vi "Initialize-panes.vi"(8 "error in (no error)":errorcluster, 10 "VI ref":refnum<vi>, 11 "UI ref. in":refnum<data-value>) -> (0 "error out":errorcluster, 3 "UI ref.":refnum<data-value>)   [LabVIEW 2013, in "CameraVision.lvlib" / "CV-UI.lvclass"]
uses:
  CV-UI.lvclass
  Panes/Pane-settings.ctl
  Panes/Pane-names.ctl
  Panes/Splitter-settings.ctl
  Panes/Splitter-names.ctl
  CV-UI.lvclass/CV-UI.ctl
  Panes/CV-Panes.lvclass
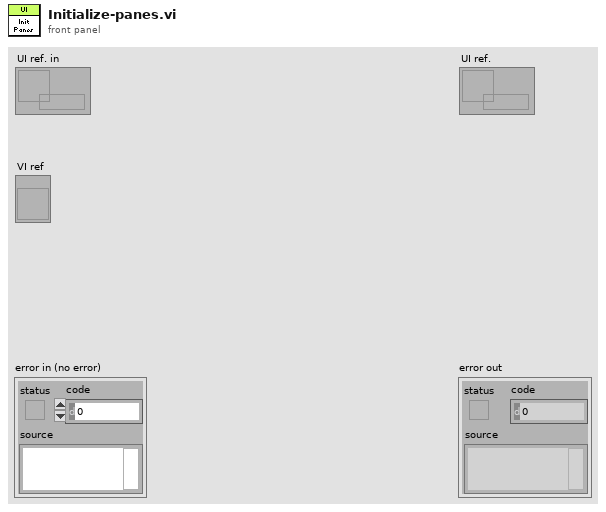
[diagram p1: front panel]
types:
  T1 = typedef "CameraVision.lvlib/CV-Panes.lvclass/Pane-settings.ctl" = cluster{"Pane-name":T2, "Startup visible?":bool, "Currently visible?":bool, "Splitters":T3[], "Pane-reference":refnum<vi>}
  T2 = typedef "CameraVision.lvlib/CV-Panes.lvclass/Pane-names.ctl" = enum16{"Toolbar", "Help bar", "Toolbar lower border", "Settings", "Displays", "Status bar upper border", "General state bar", "Information bar"}
  T3 = typedef "CameraVision.lvlib/CV-Panes.lvclass/Splitter-settings.ctl" = cluster{"Splitter-name":T4, "Position shown":i32, "Position hidden":i32, "Splitter reference":refnum<vi>}
  T4 = typedef "CameraVision.lvlib/CV-Panes.lvclass/Splitter-names.ctl" = enum16{"Upper toolbar splitter", "Help bar splitter", "Lower toolbar splitter", "Upper status bar splitter", "Lower status bar splitter", "Splitter", "Settings splitter"}
  T5 = typedef "CameraVision.lvlib/CV-Panes.lvclass/Object-reference.ctl" = refnum<data-value>
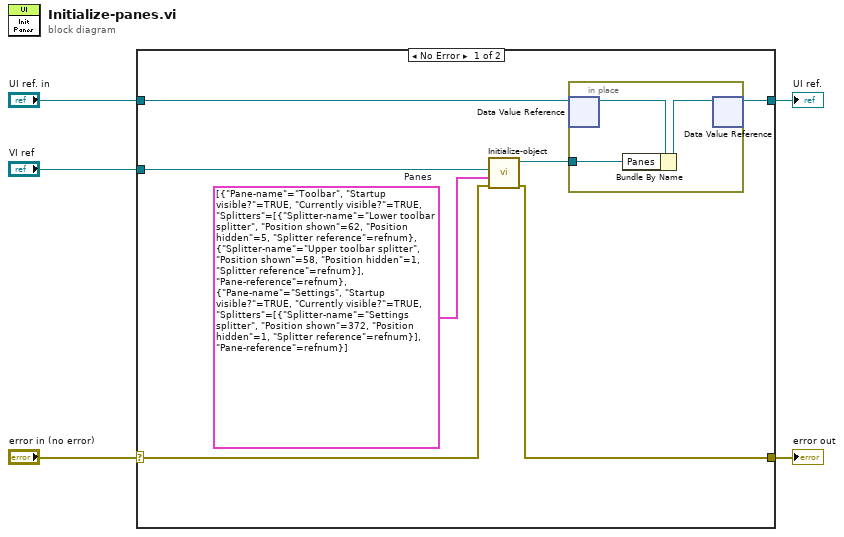
[diagram p0: block diagram]
diagram:
  n1 = case shown="No Error" "error in (no error)" {
    selector: "error in (no error)" -> [w7 w17]
    tunnel: [w6 w17] -> w4
    tunnel: [w11 w16] -> w2
    tunnel: "UI ref. in" -> [w12 w16]
    tunnel: "VI ref" -> [w9 _]
    frame No Error {
      w10 = T1[] [{"Pane-name"=enum."Toolbar", "Startup visible?"=TRUE, "Currently visible?"=TRUE, "Splitters"=[{"Splitter-name"=enum."Lower toolbar splitter", "Position shown"=62, "Position hidden"=5, "Splitter reference"=refnum}, {"Splitter-name"=enum."Upper toolbar splitter", "Position shown"=58, "Position hidden"=1, "Splitter reference"=refnum}], "Pane-reference"=refnum}, {"Pane-name"=enum."Settings", "Startup visible?"=TRUE, "Currently visible?"=TRUE, "Splitters"=[{"Splitter-name"=enum."Settings splitter", "Position shown"=372, "Position hidden"=1, "Splitter reference"=refnum}], "Pane-reference"=refnum}]  # Panes
      n2 = call "Initialize-object.vi"("error in (no error)"=w7, "Panes settings"=w10, "VI Reference"=w9) -> ("error out"=w6:errorcluster, "Panes out"=w8:T5)  [unwired: 7 in]
      n3 = in-place {
        in-place-border: w8 -> [w13]
        n4 = in-place-dvr #1(w12) -> (w15:refnum<class "CV-UI.lvclass">)  [unwired: 1 out]
        n5 = Bundle By Name(cluster=w15, "Panes"=w13) -> (w14:refnum<class "CV-UI.lvclass">)
        n6 = in-place-dvr #1(w14) -> (w11:refnum<data-value>)  [unwired: 1 out]
      }
    }
    frame Error {
    }
  }
  "error out" <- w4
  "UI ref." <- w2
